vi "ToKnob.vi"(8 "error in":errorcluster, 11 "Generic":refnum<class "Generic.lvclass">) -> (0 "error out":errorcluster, 3 "Knob out":refnum<class "Knob.lvclass">)   [LabVIEW 2014, in "Knob.lvclass"]
uses:
  Knob.lvclass
  Generic/Generic.lvclass
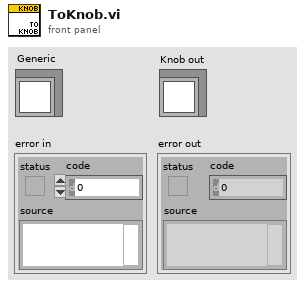
[diagram p1: front panel]
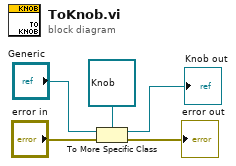
[diagram p0: block diagram]
diagram:
  n1 = To More Specific Class(target class=refnum<class "Knob.lvclass"> refnum ("Knob in"), reference="Generic", error in="error in") -> (specific class reference=→"Knob out":refnum<class "Knob.lvclass">, error out=→"error out":errorcluster)
